vi "load asynchronous call.vi"   [LabVIEW 2013, in "NISE Tools Drop Templates.lvlib"]
uses:
  NISE Tools Drop Templates.lvlib
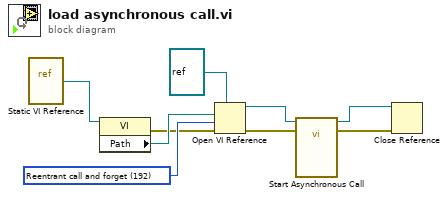
[diagram p0: block diagram]
diagram:
  w9 = 192 items=["Prepare to call and forget"=128, "Prepare to call and collect"=256, "Reentrant call and forget"=192, "Reentrant call and collect"=320] ("VI Server Options")
  n1 = vi-ref "Static VI Reference"() -> ("vi reference"=w1:refnum<vi>)
  n2 = property class="VI"(reference=w1) -> (error out=w7:errorcluster, "Path"=w8:path)  [unwired: 1 in, 1 out]
  n3 = Open VI Reference(type specifier VI Refnum (for type only)=refnum<vi> refnum, vi path=w8, options=w9, error in (no error)=w7) -> (vi reference=w5:refnum<vi>, error out=w6:errorcluster)  [unwired: 2 in]
  n4 = call-by-ref "Start Asynchronous Call"(reference=w5, error in=w6) -> (reference out=w2:refnum<vi>, error out=w3:errorcluster)  [unwired: 12 in]
  n5 = Close Reference(reference=w2, error in (no error)=w3) -> ()  [unwired: 1 out]
